vi "ep_Delete Phase N.vi"(6 "channel":T1, 8 "error in (no error)":errorcluster, 11 "spectra in":T2(array[cluster])) -> (0 "error out":errorcluster, 3 "spectra out":T2(array[cluster]))   [LabVIEW 2014, in "NI_EP_Power Quality.lvlib"]
uses:
  <vilib>/addons/Electrical Power/PQ/NI_EP_Power Quality.lvlib
  <vilib>/addons/Electrical Power/PQ/Common/Controls/ep_AI Data Channel.ctl
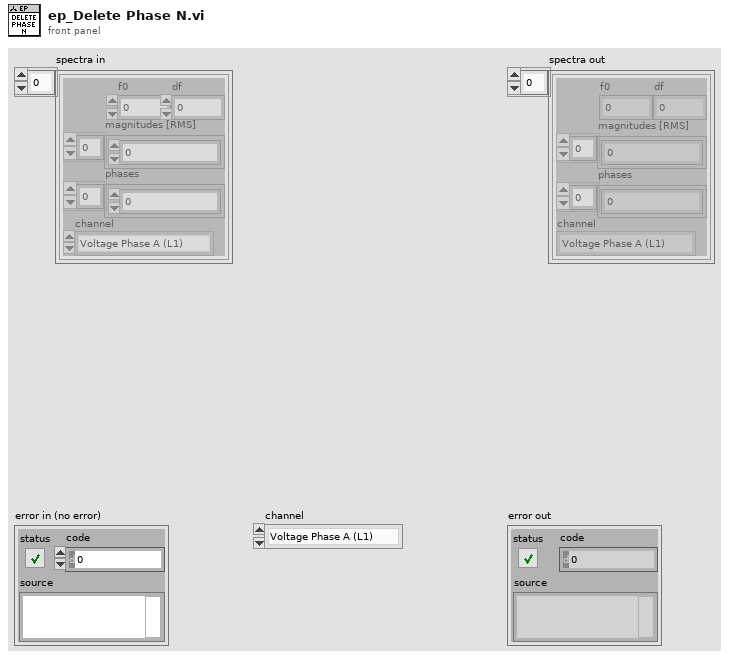
[diagram p1: front panel]
types:
  T1 = typedef "NI_EP_Power Quality.lvlib/ep_AI Data Channel.ctl" = enum16{"Voltage Phase A (L1)", "Voltage Phase B (L2)", "Voltage Phase C (L3)", "Voltage Phase N (Neutral)", "Current Phase A (L1)", "Current Phase B (L2)", "Current Phase C (L3)", "Current Phase N (Neutral)"}
  T2 = cluster{"f0":dbl, "df":dbl, "magnitudes [RMS]":dbl[], "phases":dbl[], "channel":T1}[]
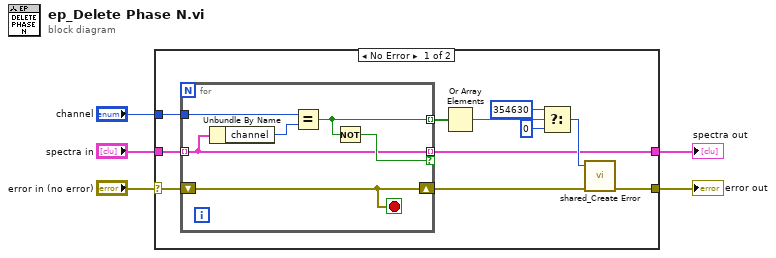
[diagram p0: block diagram]
diagram:
  n1 = case shown="No Error" "error in (no error)" {
    selector: "error in (no error)" -> [w7 w23]
    tunnel: "spectra in" -> [w10 w24]
    tunnel: [w9 w24] -> w4
    tunnel: [w8 w23] -> w3
    tunnel: "channel" -> [w6 _]
    frame No Error {
      n2 = for {
        tunnel: w10 -> [w17] mode=indexing
        shift-right: [w19] -> w11
        shift-left: w7 -> [w19]
        tunnel: w6 -> [w21]
        tunnel: [w22] -> w16 mode=indexing
        tunnel: [w17] -> w9 mode=indexing if=w20
        stop <- w19 stop-if-true
        n3 = Unbundle By Name(w17) -> ("channel"=w18:T1)
        n4 = Equal?(x=w21, y=w18) -> (x = y?=w22:bool)
        n5 = Not(x=w22) -> (.not. x?=w20:bool)
      }
      n6 = Or Array Elements(Boolean array=w16) -> (logical OR=w12:bool)
      n7 = Select(t=354630 ("error code (0)"), s=w12, f=0) -> (s? t:f=w15:i32)
      n8 = call <vilib>:"shared_Create Error.vi"("error in (no error)"=w11, "error code (0)"=w15) -> ("error out"=w8:errorcluster)  [unwired: 9 in]
    }
    frame Error {
    }
  }
  "spectra out" <- w4
  "error out" <- w3
